vi "Convert Device Units to Acceleration (FW7).vi"(9 "Microstep Size (0)":dbl, 10 "Units (0: device acceleration units)":u16(ring) items=["device acceleration units", "microns per second squared", "millimeters per second squared", "inches per second squared", "degrees per second squared"], 11 "Device Acceleration (0)":i64) -> (3 "Acceleration":dbl)   [LabVIEW 2018, in "Zaber A Series.lvlib"]
doc: "Helper to convert device-specific units of acceleration to standard units.\n\nSelect a unit and enter an a device's acceleration quantity. The output will be the acceleration converted to the selected unit.\n\nIf you select a unit other than device units, you must also provide the Microstep Size conversion factor from microsteps to micrometers, which can be found in your device manual."
uses:
  Zaber A Series.lvlib
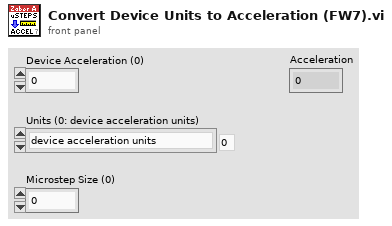
[diagram p1: front panel]
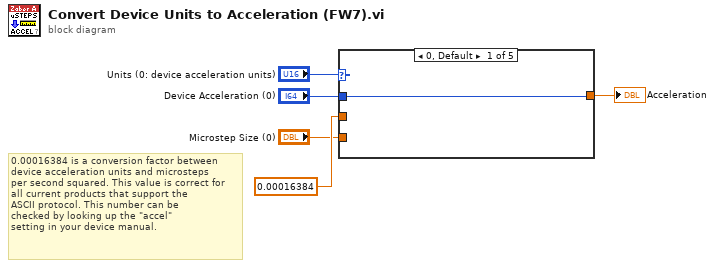
[diagram p0: block diagram]
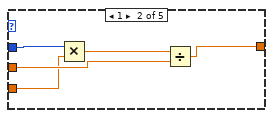
[diagram p2: hidden frame]
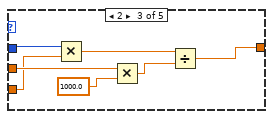
[diagram p3: hidden frame]
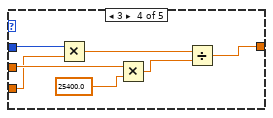
[diagram p4: hidden frame]
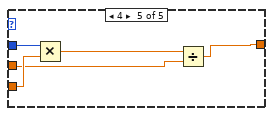
[diagram p5: hidden frame]
diagram:
  # "0.00016384 is a conversion factor between \ndevice acceleration units and microsteps \nper second squared. This value is correct for\nall current products that support the\nASCII protocol. This number can be \nchecked by looking up the \"accel\"\nsetting in your device manual."
  n1 = case shown="0, Default" "Units (0: device acceleration units)" {
    tunnel: 0.00016384 ("Acceleration Constant (0.00016384)") -> [_ w11 w15 w21 w27]
    tunnel: "Microstep Size (0)" -> [_ w7 w12 w19 w28]
    tunnel: [w6 w9 w18 w25 w26] -> w1
    tunnel: "Device Acceleration (0)" -> [w6 w8 w17 w24 w29]
    frame 0, Default {
    }
    frame 1 {
      n2 = Multiply(x=w8, y=w7) -> (x*y=w10:dbl)
      n3 = Divide(x=w10, y=w11) -> (x/y=w9:dbl)
    }
    frame 2 {
      n4 = Multiply(x=w17, y=w12) -> (x*y=w13:dbl)
      n5 = Multiply(x=w15, y=1000.0) -> (x*y=w14:dbl)
      n6 = Divide(x=w13, y=w14) -> (x/y=w18:dbl)
    }
    frame 3 {
      n7 = Multiply(x=w24, y=w19) -> (x*y=w23:dbl)
      n8 = Multiply(x=w21, y=25400.0) -> (x*y=w20:dbl)
      n9 = Divide(x=w23, y=w20) -> (x/y=w25:dbl)
    }
    frame 4 {
      n10 = Multiply(x=w29, y=w28) -> (x*y=w30:dbl)
      n11 = Divide(x=w30, y=w27) -> (x/y=w26:dbl)
    }
  }
  "Acceleration" <- w1
